vi "Stage 3.1 Getting the hardware out.vi"() -> ()   [LabVIEW 2020]
uses:
  <vilib>/measure/matone.llb/Extract Single Tone Information 1 Chan.vi
  <vilib>/measure/NI_MAPro.lvlib
panel:
  out "data":waveform(dbl)
  out "error out Hardware":errorcluster
  in  "Addition signal to remove (0) [s]":dbl
  out "Pulse":dbl
  out "Filtered":waveform(dbl)(graph)
  in  "Samples size (10) [s]":i32=10
  out "Raw":waveform(dbl)(graph)
  in  "Stop":bool
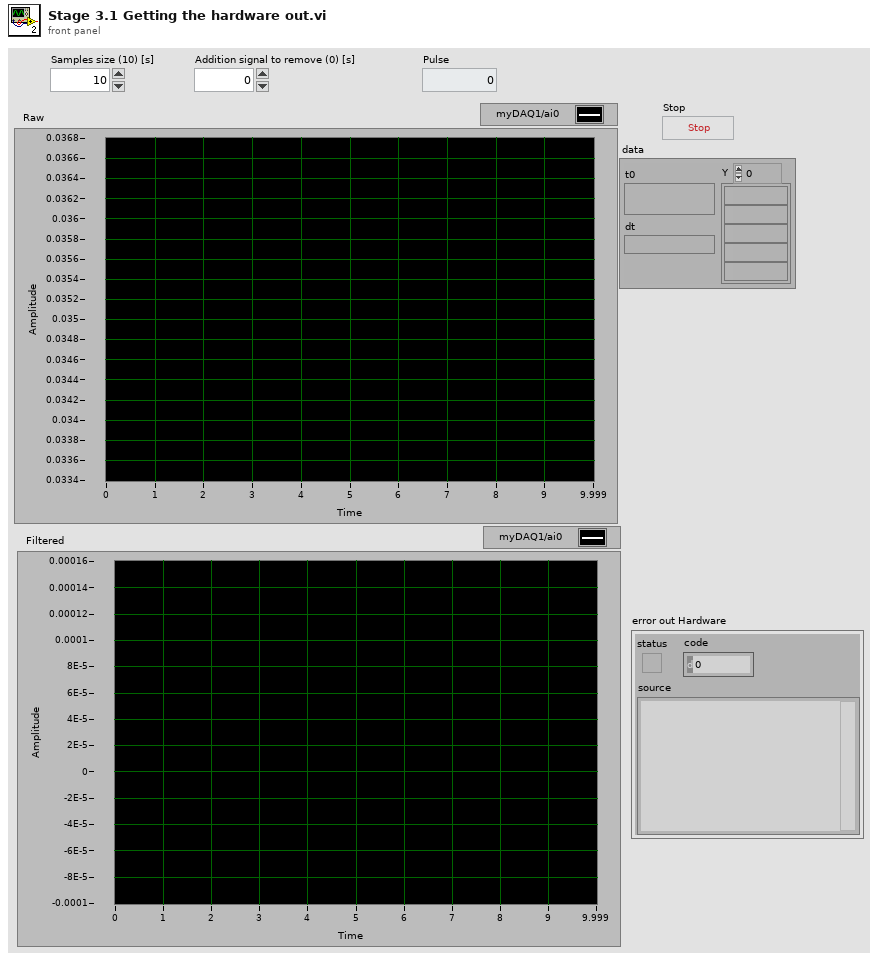
[diagram p1: front panel]
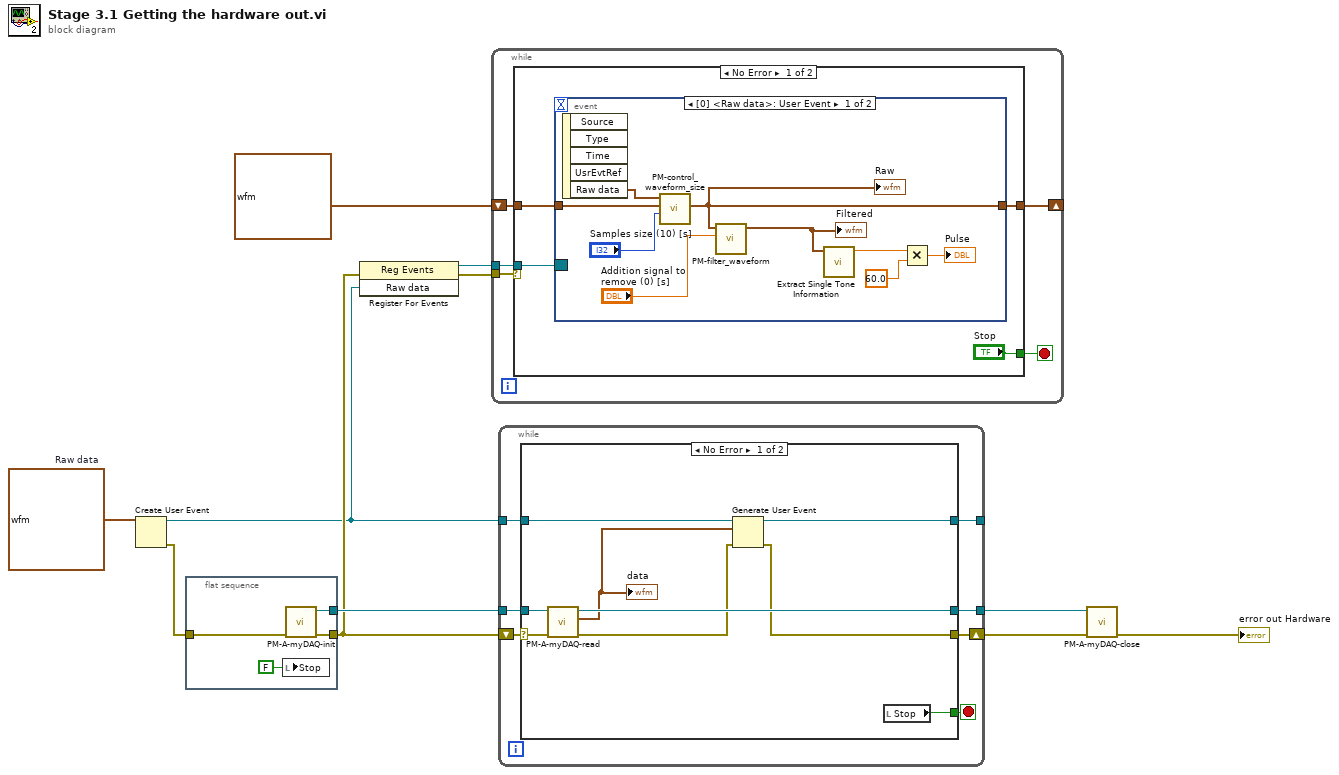
[diagram p0: block diagram]
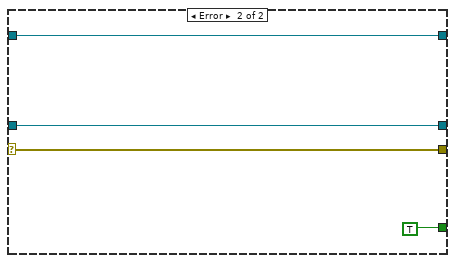
[diagram p2: hidden frame]
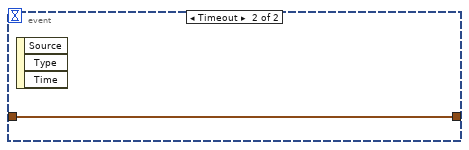
[diagram p3: hidden frame]
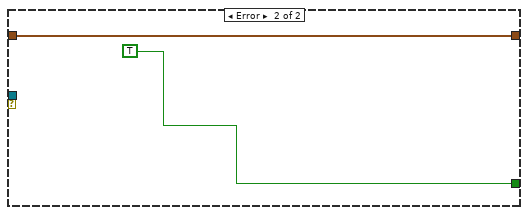
[diagram p4: hidden frame]
diagram:
  w7 = waveform(dbl) {"t0"=timestamp(0 s since 1904-01-01), "dt"=1.0, "Y"=[]}  # Raw data
  n1 = Create User Event(user event datatype=w7) -> (user event=w4:refnum<user-event>, error out=w6:errorcluster)  [unwired: 1 in]
  n2 = flat-sequence {
    tunnel: [w15] -> w8
    tunnel: [w14] -> w5
    tunnel: w6 -> [w12]
    frame #0 {
      n3 = local write "Stop"(FALSE ("Stop")) -> ()
      n4 = call "PM-A-myDAQ-init.vi"("error in"=w12) -> ("error out"=w14:errorcluster, "Refnum out"=w15:refnum<k21>)  [unwired: 9 in]
    }
  }
  n5 = register-events(error in=w5, w4) -> (reference out=w2:refnum<event-registration>, error out=w3:errorcluster)  [unwired: 1 in]
  n6 = while {
    shift-right: [w18] -> _
    shift-left: waveform(dbl) {"t0"=timestamp(0 s since 1904-01-01), "dt"=0.0, "Y"=[]} ("data") -> [w19]
    tunnel: w3 -> [w17]
    tunnel: w2 -> [w16]
    stop <- w20 stop-if-true
    n7 = case shown="No Error" w17 {
      tunnel: ["Stop" TRUE ("Stop")] -> w20
      tunnel: w19 -> [w23 w35]
      tunnel: [w22 w35] -> w18
      tunnel: w16 -> [w21 _]
      frame No Error {
        n8 = event shown="[0] <Raw data>: User Event" {
          selector: w21 -> [_ _]
          dyn-events: _ -> [_ _]
          timeout: _ -> [_ _]
          tunnel: w23 -> [w32 w34]
          tunnel: [w31 w34] -> w22
          event User Event {
            n9 = event-data() -> ("Raw data"=w25:waveform(dbl))  [unwired: 1 in, 4 out]
            n10 = call "PM-control_waveform_size.vi"("Samples s"="Samples size (10) [s]", "old waveform"=w32, "New waveform"=w25) -> ("waveform"=w31:waveform(dbl))  [unwired: 8 in]
            "Raw" <- w31
            n11 = call "PM-filter_waveform.vi"("Addition signal to remove (0) [s]"="Addition signal to remove (0) [s]", "waveform in"=w31) -> ("waveform out"=w30:waveform(dbl))  [unwired: 8 in, 1 out]
            "Filtered" <- w30
            n12 = call-poly <vilib>:"Extract Single Tone Information.vi"("time signal in"=w30) -> ("detected frequency"=w29:dbl)  [unwired: 5 in, 5 out]
            n13 = Multiply(x=w29, y=60.0) -> (x*y=→"Pulse":dbl)
          }
          event Timeout {
            n14 = event-data() -> ()  [unwired: 1 in, 3 out]
          }
        }
      }
      frame Error {
      }
    }
  }
  n15 = while {
    tunnel: w8 -> [w43]
    tunnel: [w41] -> w9
    shift-right: [w40] -> w10
    shift-left: w5 -> [w42]
    tunnel: w4 -> [w38]
    tunnel: [w37] -> _
    stop <- w39 stop-if-true
    n16 = case shown="No Error" w42 {
      selector: w42 -> [w51 w55]
      tunnel: w43 -> [w52 w54]
      tunnel: [w50 w54] -> w41
      tunnel: [w45 w55] -> w40
      tunnel: [w49 TRUE ("Stop")] -> w39
      tunnel: w38 -> [w48 w53]
      tunnel: [w44 w53] -> w37
      frame No Error {
        n17 = call "PM-A-myDAQ-read.vi"("error in (no error)"=w51, "Refnum in"=w52) -> ("error out"=w46:errorcluster, "data"=w47:waveform(dbl), "Refnum out"=w50:refnum<k21>)  [unwired: 7 in]
        "data" <- w47
        n18 = Generate User Event(user event=w48, event data cluster=w47, error in=w46) -> (user event out=w44:refnum<user-event>, error out=w45:errorcluster)  [unwired: 1 in]
        n19 = local read "Stop"() -> (w49:bool)
      }
      frame Error {
      }
    }
  }
  n20 = call "PM-A-myDAQ-close.vi"("error in (no error)"=w10, "Refnum in"=w9) -> ("error out"=→"error out Hardware":errorcluster)  [unwired: 9 in]
